vi "Start.vi"(8 "error in (no error)":errorcluster, 10 "Message in":refnum<class "StartMessage.lvclass">, 11 "DAQCascade512II in":refnum<class "DAQCascade512II.lvclass">) -> (0 "error out":errorcluster, 3 "DAQCascade512II out":refnum<class "DAQCascade512II.lvclass">)   [LabVIEW 2012, in "DAQCascade512II.lvclass"]
doc: "This member function is called when the statemachine in the run.vi receives an 'start' command. It relays the message to all observers of the component.\n\nOverride this member function in your derived class if you need additional start functionality (but don't forget to call the parent method)."
uses:
  DAQCascade512II.lvclass
  <vilib>/Distrio/Murmex/StartMessage/StartMessage.lvclass
  <vilib>/Distrio/Murmex/Murmex/Murmex.lvclass
  DAQCascade512II.lvclass/DAQCascade512II.ctl
panel:
  out "Display Title":string
  in  "save images?":bool
  in  "stop":bool
  # "This member function is called when the statemachine in the run.vi receives an 'start' command. It relays the message to all observers of the component.\n\nOverride this member function in your derived class if you need additional start functionality (but don't forget to call the parent method)."
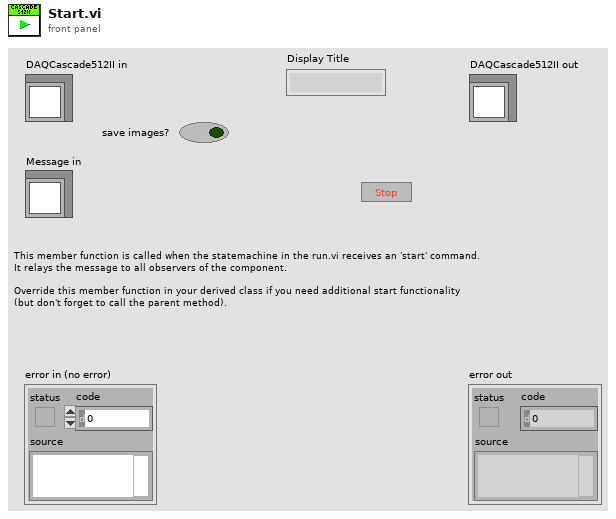
[diagram p1: front panel]
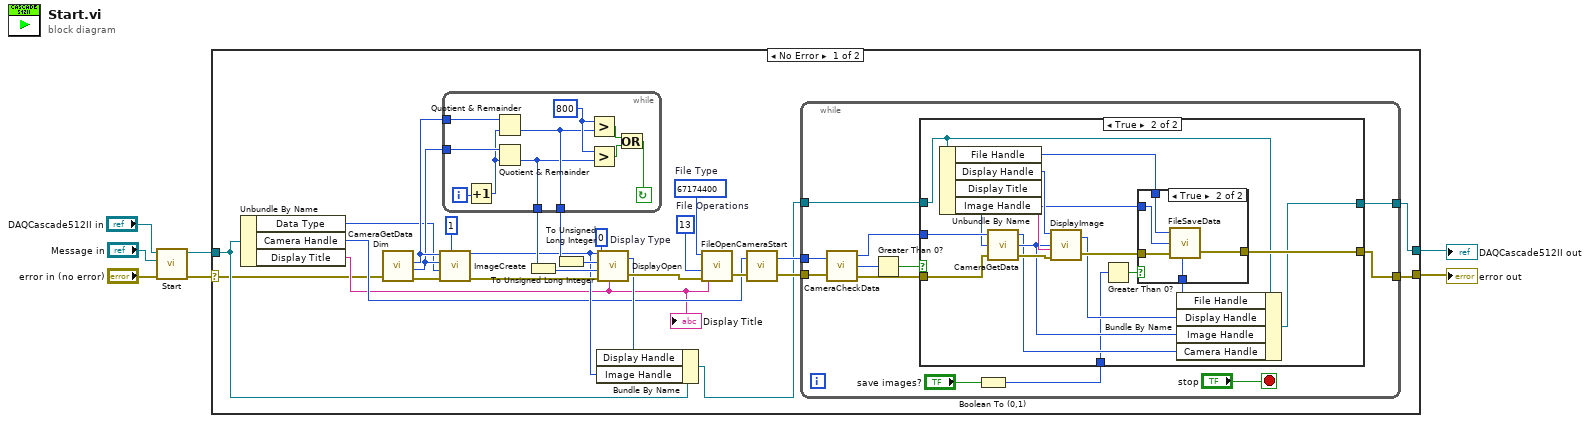
[diagram p0: block diagram]
diagram:
  n1 = call-parent "Start.vi"("error in (no error)"="error in (no error)", "Message in"="Message in", "Murmex in"="DAQCascade512II in") -> ("error out"=w4:errorcluster, "Murmex out"=w2:refnum<class "DAQCascade512II.lvclass">)  [unwired: 7 in]
  n2 = case shown="No Error" w4 {
    selector: w4 -> [w8 w81]
    tunnel: [w13 w82] -> w3
    tunnel: w2 -> [w15 w82]
    tunnel: [w12 w81] -> w1
    frame No Error {
      w22 = 67174400  # File Type
      w21 = 13  # File Operations
      w24 = u32 0  # Display Type
      n3 = Unbundle By Name(w15) -> ("Data Type"=w10:u32, "Camera Handle"=w11:u32, "Display Title"=w9:string)
      "Display Title" <- w9
      n4 = call <userlib>:"CameraGetDataDim.vi"("error in"=w8) -> ("Xdim"=w30:u32, "Ydim"=w29:u32, "error out"=w31:errorcluster)  [unwired: 1 in, 1 out]
      n5 = call <userlib>:"ImageCreate.vi"("X dimension"=w30, "Y dimension"=w29, "Data Type"=w10, "error in"=w31, "Number Of Frames"=u32 1) -> ("Image Handle"=w17:u32)  [unwired: 1 out]
      n6 = while {
        tunnel: w30 -> [w80]
        tunnel: w29 -> [w79]
        tunnel: [w72] -> w25
        tunnel: [w71] -> w28
        i -> [w78]
        stop <- w73 continue-if-true
        w76 = u32 800 ("x")
        n7 = Increment(x=w78) -> (x+1=w77:i32)
        n8 = Quotient & Remainder(x=w80, y=w77) -> (floor(x/y)=w72:u32)  [unwired: 1 out]
        n9 = Quotient & Remainder(x=w79, y=w77) -> (floor(x/y)=w71:u32)  [unwired: 1 out]
        n10 = Greater?(x=w76, y=w72) -> (0:w74:bool)
        n11 = Greater?(x=w76, y=w71) -> (0:w75:bool)
        n12 = Or(x=w74, y=w75) -> (x .or. y?=w73:bool)
      }
      n13 = To Unsigned Long Integer(number=w28) -> (unsigned 32bit integer=w27:u32)
      n14 = To Unsigned Long Integer(number=w25) -> (unsigned 32bit integer=w26:u32)
      n15 = call <userlib>:"DisplayOpen.vi"("Display Title"=w9, "Image Handle"=w17, "error in"=w31, "Display Height"=w27, "Display Width"=w26, "Display Type"=w24) -> ("error out"=w23:errorcluster, "Display Handle"=w16:u32)
      n16 = Bundle By Name(cluster=w15, "Display Handle"=w16, "Image Handle"=w17) -> (w14:refnum<class "DAQCascade512II.lvclass">)
      n17 = call <userlib>:"FileOpen.vi"("error in"=w23, "File Operations"=w21, "FileName"=w9, "File Type"=w22) -> ("error out"=w20:errorcluster)  [unwired: 1 out]
      n18 = call <userlib>:"CameraStart.vi"("error in"=w20, "Camera Handle"=w11) -> ("error out"=w18:errorcluster, "Camera Handle"=w19:u32)
      n19 = while {
        tunnel: w19 -> [w44]
        tunnel: w18 -> [w41]
        tunnel: w14 -> [w38]
        tunnel: [w36] -> w13
        tunnel: [w35] -> w12
        stop <- "stop" stop-if-true
        n20 = call <userlib>:"CameraCheckData.vi"("Camera Handle"=w44, "error in"=w41) -> ("Camera Handle"=w39:u32, "Number Of Frames Available"=w43:i32, "error out"=w37:errorcluster)
        n21 = Greater Than 0?(x=w43) -> (x > 0?=w42:bool)
        n22 = Boolean To (0,1)(Boolean="save images?") -> (0, 1=w33:i16)
        n23 = case shown="True" w42 {
          tunnel: w39 -> [_ w63]
          tunnel: w38 -> [w46 w54]
          tunnel: w37 -> [w45 w62]
          tunnel: [w46 w49] -> w36
          tunnel: [w45 w55] -> w35
          tunnel: w33 -> [_ w48]
          frame False {
          }
          frame True {
            n24 = Unbundle By Name(w54) -> ("File Handle"=w58:u32, "Display Handle"=w59:u32, "Display Title"=w60:string, "Image Handle"=w57:u32)
            n25 = call <userlib>:"CameraGetData.vi"("error in"=w62, "Data Handle"=w57, "Camera Handle"=w63) -> ("error out"=w61:errorcluster, "Data Handle"=w51:u32, "Camera Handle"=w50:u32)
            n26 = call <userlib>:"DisplayImage.vi"("error in"=w61, "Title"=w60, "Image Handle"=w51, "Display Handle"=w59) -> ("error out"=w56:errorcluster, "Display Handle"=w52:u32)
            n27 = Greater Than 0?(x=w48) -> (x > 0?=w47:bool)
            n28 = case shown="True" w47 {
              tunnel: w58 -> [w64 w70]
              tunnel: w57 -> [_ w69]
              tunnel: w56 -> [w65 w68]
              tunnel: [w65 w67] -> w55
              tunnel: [w64 w66] -> w53
              frame False {
              }
              frame True {
                n29 = call <userlib>:"FileSaveData.vi"("error in"=w68, "Image Handle"=w69, "File Handle"=w70) -> ("error out"=w67:errorcluster, "File Handle"=w66:u32)
              }
            }
            n30 = Bundle By Name(cluster=w54, "File Handle"=w53, "Display Handle"=w52, "Image Handle"=w51, "Camera Handle"=w50) -> (w49:refnum<class "DAQCascade512II.lvclass">)
          }
        }
      }
    }
    frame Error {
    }
  }
  "error out" <- w1
  "DAQCascade512II out" <- w3
